vi "Init ref kill.vi"(7 "Action":T2=enum."Ref", 8 "Error In":errorcluster) -> (0 "Error Out":errorcluster, 3 "Messages":T1)   [LabVIEW 2017, in "Events.lvlib"]
uses:
  Events.lvlib
  Controls/Action Refs [enum].ctl
  Controls/Refs [cluster].ctl
  System Control/CTLs/Command Data [cluster].ctl
  System Control/CTLs/Commands [enum].ctl
  Controls/Error Data [cluster].ctl
  UI/Controls/Command Data [cluster].ctl
  UI/Controls/Commands [enum].ctl
  Example Module/Controls/Command Data [cluster].ctl
  Example Module/Controls/Commands [enum].ctl
  Shutter Module/Controls/Module Command Data [cluster].ctl
  Shutter Module/Controls/Module Commands [enum].ctl
  Monochromator/Controls/Command Data [cluster].ctl
  Monochromator/Controls/Commands [enum].ctl
  DAQ/Controls/Command Data [cluster].ctl
  DAQ/Controls/Commands [enum].ctl
  Scope/Controls/Command Data [cluster].ctl
  Scope/Controls/Commands [enum].ctl
  Processing/Controls/Command Data [cluster].ctl
  Processing/Controls/Commands [enum].ctl
  File IO/Controls/Command Data [cluster].ctl
  File IO/Controls/Commands [enum].ctl
  Colour Wheel/Controls/Command Data [cluster].ctl
  Colour Wheel/Controls/Commands [enum].ctl
  Example Module/Example Module.lvlib
  Shutter Module/Shutter.lvlib
  Monochromator/Monochromator.lvlib
  UI/UI.lvlib
  System Control/Main controller.lvlib
  DAQ/DAQ.lvlib
  Processing/Processing.lvlib
  Scope/Scope.lvlib
  File IO/File IO.lvlib
  Colour Wheel/Colour Wheel.lvlib
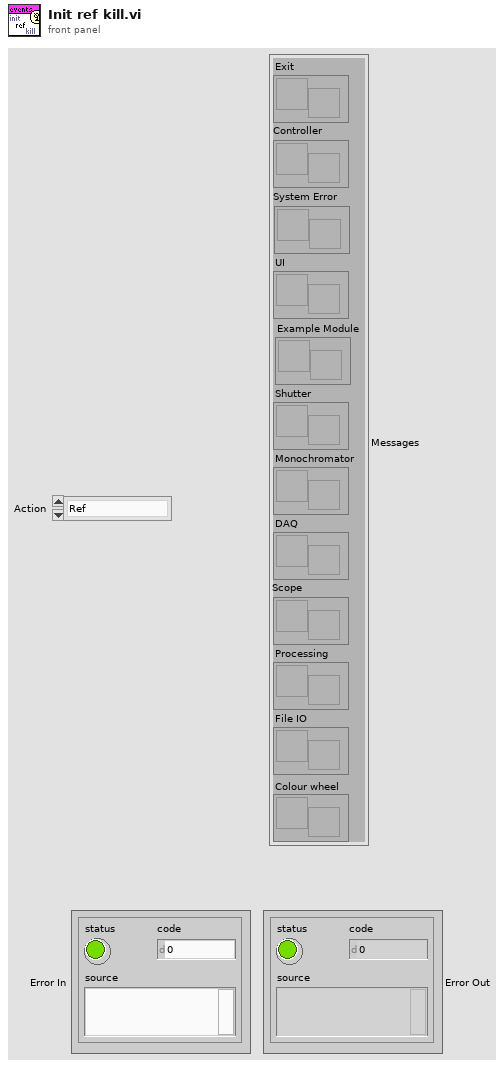
[diagram p1: front panel]
types:
  T1 = typedef "Events.lvlib/Refs [cluster].ctl" = cluster{"Exit":refnum<user-event>, "Controller":refnum<user-event>, "System Error":refnum<user-event>, "UI":refnum<user-event>, "Example Module":refnum<user-event>, "Shutter":refnum<user-event>, "Monochromator":refnum<user-event>, "DAQ":refnum<user-event>, "Scope":refnum<user-event>, "Processing":refnum<user-event>, "File IO":refnum<user-event>, "Colour wheel":refnum<user-event>}
  T2 = typedef "Events.lvlib/Action Refs [enum].ctl" = enum16{"Init", "Ref", "Kill"}
  T3 = typedef "Colour Wheel.lvlib/Command Data [cluster].ctl" = cluster{"Command":T4, "Data":variant}
  T4 = typedef "Colour Wheel.lvlib/Commands [enum].ctl" = enum16{"Start", "Move", "Get position", "Stop", "Send data"}
  T5 = typedef "Shutter.lvlib/Module Command Data [cluster].ctl" = cluster{"Command":T6, "Data":variant}
  T6 = typedef "Shutter.lvlib/Module Commands [enum].ctl" = enum16{"Start", "Move", "Return", "Stop"}
  T7 = typedef "File IO.lvlib/Command Data [cluster].ctl" = cluster{"Command":T8, "Data":variant}
  T8 = typedef "File IO.lvlib/Commands [enum].ctl" = enum16{"Start", "Stop", "Read waveform", "Write waveform", "Delete waveform", "Log error", "Write config", "Read config", "Save parameters", "Send waveform to processing", "Update file prefix"}
  T9 = typedef "Scope.lvlib/Command Data [cluster].ctl" = cluster{"Command":T10, "Data":variant}
  T10 = typedef "Scope.lvlib/Commands [enum].ctl" = enum16{"Calculate parameters", "Start", "Stop", "Send data", "Start acquisition", "Get test data", "Accumulate test data", "Average test data", "Add background voltage", "Scale TPC", "Average Pre Trigger Data", "Write to file"}
  T11 = typedef "Processing.lvlib/Command Data [cluster].ctl" = cluster{"Command":T12, "Data":variant}
  T12 = typedef "Processing.lvlib/Commands [enum].ctl" = enum16{"Start", "Stop", "Process waveform", "Scope A-B processing", "DAQ A-B processing", "DAQ-Scope Stitching", "Update Test Info"}
  T13 = typedef "DAQ.lvlib/Command Data [cluster].ctl" = cluster{"Command":T14, "Data":variant}
  T14 = typedef "DAQ.lvlib/Commands [enum].ctl" = enum16{"Calculate parameters", "Start", "Stop", "Get test data", "Accumulate test data", "Average test data", "Calculate background voltage", "Send data", "Write data to file"}
  T15 = typedef "UI.lvlib/Command Data [cluster].ctl" = cluster{"Command":T16, "Data":variant}
  T16 = typedef "UI.lvlib/Commands [enum].ctl" = enum16{"Start", "Update", "Acquisition Complete", "Stop", "Set DAQ data", "Set Scope data", "Set processing data", "Clear Graphs"}
  T17 = typedef "Monochromator.lvlib/Command Data [cluster].ctl" = cluster{"Command":T18, "Data":variant}
  T18 = typedef "Monochromator.lvlib/Commands [enum].ctl" = enum16{"Start", "Spectrum setup", "Spectrum move", "Monochromator Setup", "Move", "GetPosition", "Stop", "Send data"}
  T19 = typedef "Example Module.lvlib/Command Data [cluster].ctl" = cluster{"Command":T20, "Data":variant}
  T20 = typedef "Example Module.lvlib/Commands [enum].ctl" = enum16{"Start", "Stop", "Send config"}
  T21 = typedef "Main controller.lvlib/Command Data [cluster].ctl" = cluster{"Command":T22, "Data":variant}
  T22 = typedef "Main controller.lvlib/Commands [enum].ctl" = enum16{"Start", "Initialise Devices", "Stop", "Set DAQ data", "Set Scope data", "Set Spectrum Setup", "Spectrum Setup Complete", "Set Monochromator Setup", "Monochromator Setup Complete", "Set Monochromator data", "Set Colour Wheel Setup", "Colour Wheel Setup Complete", "Move Shutter", "Move Shutter Complete", "Collect Data", "DAQ Acquisition Complete", "Scope Acquisition Complete", "Collect Data Complete", "A-B Processing", "A-B Processing Complete", "DAQ-Scope Stitching", "DAQ-Scope Stitching Complete", "Return Shutter", "Return Shutter Complete", "Set colour wheel data", "Set all config data", "Acquire test data", "Accumulate test data", "Average test data", "All Averaging Complete", "DAQ Averaging Complete", "Scope Averaging Complete", "Finalise test data", "All Finalising Complete", "DAQ Finalising Complete", "Scope Finalising Complete", "Process test data", "End Test"}
  T23 = typedef "Events.lvlib/Error Data [cluster].ctl" = cluster{"Error":string, "Error Cluster":errorcluster}
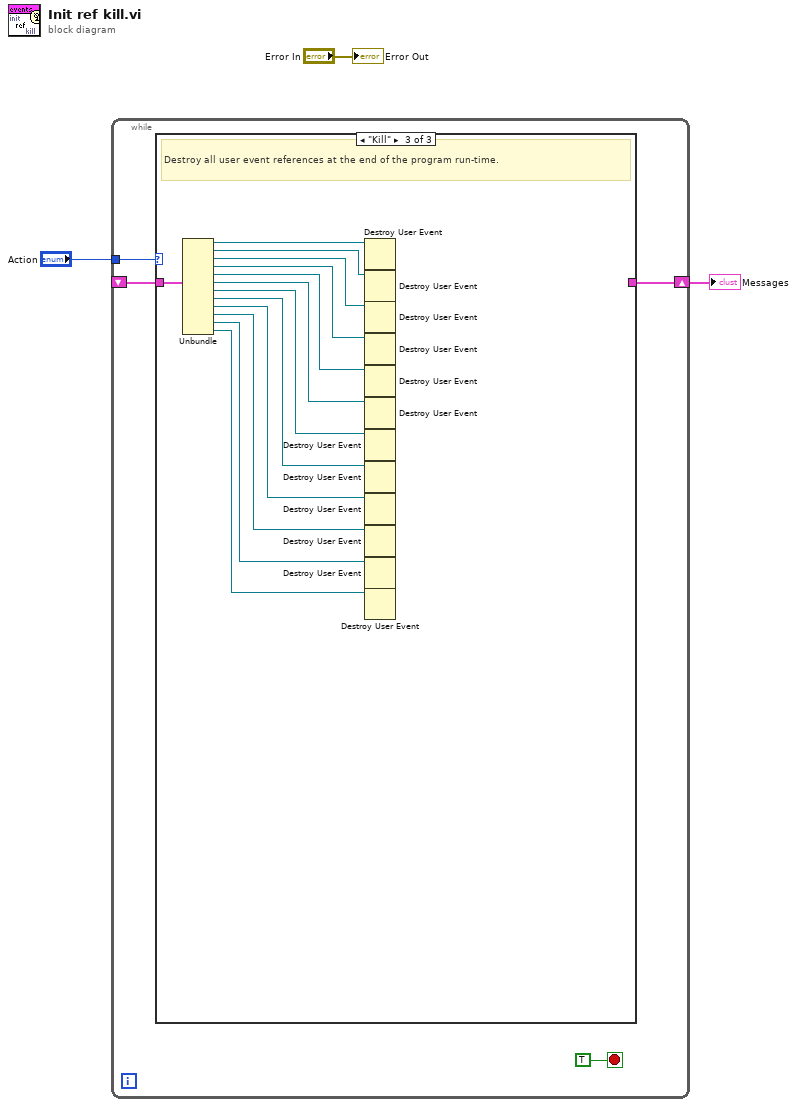
[diagram p0: block diagram]
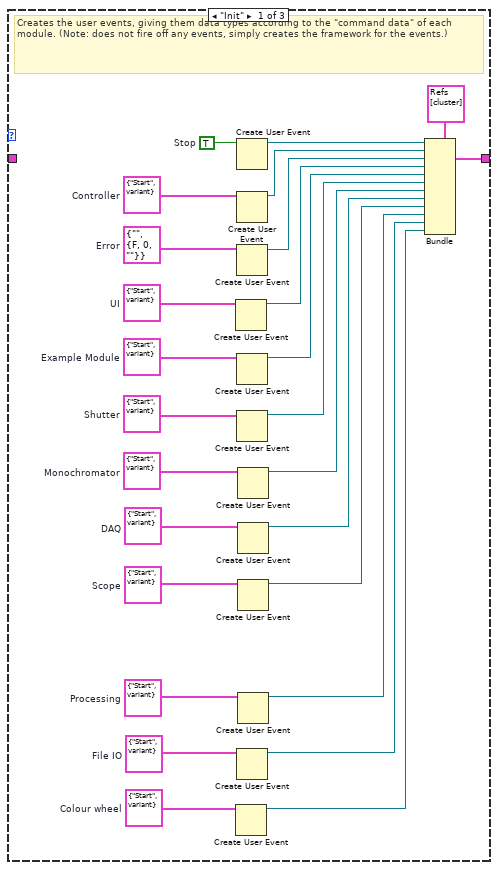
[diagram p2: hidden frame]
diagram:
  n1 = while {
    tunnel: "Action" -> [w6]
    shift-right: [w5] -> w1
    shift-left: _ -> [w4]
    stop <- TRUE stop-if-true
    n2 = case shown="\"Kill\"" w6 {
      tunnel: [w31 w34 _] -> w5
      tunnel: w4 -> [_ w34 w47]
      frame "Init" {
        w9 = T3 {"Command"=enum."Start", "Data"=variant}  # Colour wheel
        w10 = T5 {"Command"=enum."Start", "Data"=variant}  # Shutter
        w11 = T7 {"Command"=enum."Start", "Data"=variant}  # File IO
        w12 = T9 {"Command"=enum."Start", "Data"=variant}  # Scope
        w13 = T11 {"Command"=enum."Start", "Data"=variant}  # Processing
        w14 = T13 {"Command"=enum."Start", "Data"=variant}  # DAQ
        w15 = T15 {"Command"=enum."Start", "Data"=variant}  # UI
        w16 = T17 {"Command"=enum."Start", "Data"=variant}  # Monochromator
        w17 = T19 {"Command"=enum."Start", "Data"=variant}  # Example Module
        w28 = T21 {"Command"=enum."Start", "Data"=variant}  # Controller
        w29 = T23 {"Error"="", "Error Cluster"={"status"=FALSE, "code"=0, "source"=""}}  # Error
        w33 = TRUE  # Stop
        # "Creates the user events, giving them data types according to the \"command data\" of each module. (Note: does not fire off any events, simply creates the framework for the events.)"
        n3 = Create User Event(user event datatype=w15) -> (user event=w24:refnum<user-event>)  [unwired: 1 in, 1 out]
        n4 = Create User Event(user event datatype=w9) -> (user event=w8:refnum<user-event>)  [unwired: 1 in, 1 out]
        n5 = Create User Event(user event datatype=w33) -> (user event=w32:refnum<user-event>)  [unwired: 1 in, 1 out]
        n6 = Create User Event(user event datatype=w28) -> (user event=w22:refnum<user-event>)  [unwired: 1 in, 1 out]
        n7 = Create User Event(user event datatype=w29) -> (user event=w23:refnum<user-event>)  [unwired: 1 in, 1 out]
        n8 = Create User Event(user event datatype=w17) -> (user event=w25:refnum<user-event>)  [unwired: 1 in, 1 out]
        n9 = Create User Event(user event datatype=w10) -> (user event=w26:refnum<user-event>)  [unwired: 1 in, 1 out]
        n10 = Create User Event(user event datatype=w11) -> (user event=w18:refnum<user-event>)  [unwired: 1 in, 1 out]
        n11 = Create User Event(user event datatype=w16) -> (user event=w27:refnum<user-event>)  [unwired: 1 in, 1 out]
        n12 = Create User Event(user event datatype=w14) -> (user event=w21:refnum<user-event>)  [unwired: 1 in, 1 out]
        n13 = Create User Event(user event datatype=w12) -> (user event=w20:refnum<user-event>)  [unwired: 1 in, 1 out]
        n14 = Create User Event(user event datatype=w13) -> (user event=w19:refnum<user-event>)  [unwired: 1 in, 1 out]
        n15 = Bundle(cluster=T1 {"Exit"=refnum, "Controller"=refnum, "System Error"=refnum, "UI"=refnum, "Example Module"=refnum, "Shutter"=refnum, "Monochromator"=refnum, "DAQ"=refnum, "Scope"=refnum, "Processing"=refnum, "File IO"=refnum, "Colour wheel"=refnum}, "Exit"=w32, "Controller"=w22, "System Error"=w23, "UI"=w24, "Example Module"=w25, "Shutter"=w26, "Monochromator"=w27, "DAQ"=w21, "Scope"=w20, "Processing"=w19, "File IO"=w18, "Colour wheel"=w8) -> (w31:T1)
      }
      frame "Ref" {
        # "Gives a reference to the events initialised in the Init case, so that modules can register (i.e. start listening for) the events."
      }
      frame "Kill" {
        # "Destroy all user event references at the end of the program run-time."
        n16 = Unbundle(w47) -> ("Exit"=w46:refnum<user-event>, "Controller"=w45:refnum<user-event>, "System Error"=w44:refnum<user-event>, "UI"=w43:refnum<user-event>, "Example Module"=w42:refnum<user-event>, "Shutter"=w41:refnum<user-event>, "Monochromator"=w40:refnum<user-event>, "DAQ"=w39:refnum<user-event>, "Scope"=w38:refnum<user-event>, "Processing"=w37:refnum<user-event>, "File IO"=w36:refnum<user-event>, "Colour wheel"=w35:refnum<user-event>)
        n17 = Destroy User Event(user event=w46) -> ()  [unwired: 1 in, 1 out]
        n18 = Destroy User Event(user event=w45) -> ()  [unwired: 1 in, 1 out]
        n19 = Destroy User Event(user event=w44) -> ()  [unwired: 1 in, 1 out]
        n20 = Destroy User Event(user event=w43) -> ()  [unwired: 1 in, 1 out]
        n21 = Destroy User Event(user event=w42) -> ()  [unwired: 1 in, 1 out]
        n22 = Destroy User Event(user event=w41) -> ()  [unwired: 1 in, 1 out]
        n23 = Destroy User Event(user event=w40) -> ()  [unwired: 1 in, 1 out]
        n24 = Destroy User Event(user event=w39) -> ()  [unwired: 1 in, 1 out]
        n25 = Destroy User Event(user event=w38) -> ()  [unwired: 1 in, 1 out]
        n26 = Destroy User Event(user event=w37) -> ()  [unwired: 1 in, 1 out]
        n27 = Destroy User Event(user event=w36) -> ()  [unwired: 1 in, 1 out]
        n28 = Destroy User Event(user event=w35) -> ()  [unwired: 1 in, 1 out]
      }
    }
  }
  "Messages" <- w1
  "Error Out" <- "Error In"
